vi "GetStringFromRing.vi"(8 "error in (no error)":errorcluster, 11 "Ring Reference":refnum<vi>) -> (0 "error out":errorcluster, 3 "String":string)   [LabVIEW 2017, in "JKI Simple Localization.lvlib"]
uses:
  API/JKI Simple Localization.lvlib
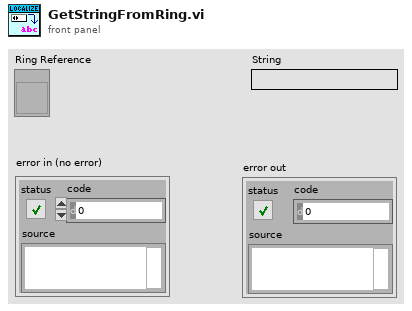
[diagram p1: front panel]
types:
  T1 = typedef "LVStringsAndValuesArrayTypeDef_U16.ctl" = cluster{"String":string, "Value":u16}[]
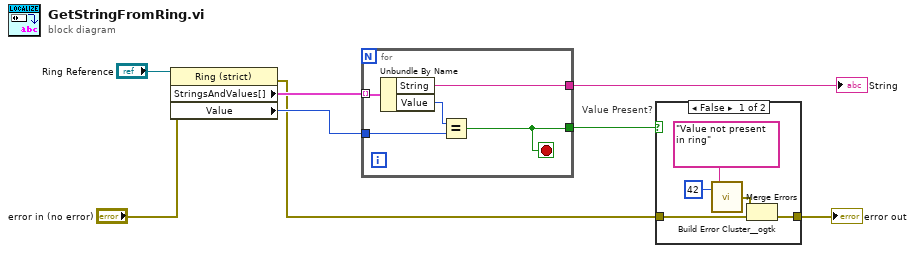
[diagram p0: block diagram]
diagram:
  n1 = property on="Property Node" class="Ring (strict)"(reference="Ring Reference", error in="error in (no error)") -> (error out=w2:errorcluster, "StringsAndValues[]"=w8:T1, "Value"=w7:u16)  [unwired: 1 out]
  n2 = for {
    tunnel: w8 -> [w13] mode=indexing
    tunnel: w7 -> [w11]
    tunnel: [w10] -> w3
    tunnel: [w9] -> w6
    stop <- w10 stop-if-true
    n3 = Unbundle By Name(w13) -> ("String"=w9:string, "Value"=w12:u16)
    n4 = Equal?(x=w12, y=w11) -> (x = y?=w10:bool)
  }
  "String" <- w6
  n5 = case "Value Present?" shown="False" w3 {
    tunnel: w2 -> [w14 w19]
    tunnel: [w15 w19] -> w1
    frame False {
      n6 = call <userlib>:"Build Error Cluster__ogtk.vi"("String to Prepend to source (\"\")"="Value not present in ring" ("String to Prepend to source (\"\")"), "code"=42) -> ("error out"=w16:errorcluster)
      n7 = Merge Errors(w16, w14) -> (w15:errorcluster)
    }
    frame True {
    }
  }
  "error out" <- w1
